vi "LTE Configure Common.vi"(0 "RFmx Handle In":refnum<k21>, 1 "Selector String":string, 5 "Common Configuration":T1={"Center Frequency (Hz)"=1000000000.0, "Reference Level (dBm)"=0.0, "External Attenuation (dB)"=0.0, "Trigger Enabled"=TRUE, "Digital Trigger Source"="PXI_Trig0", "Trigger Delay (s)"=0.0, "Selected Ports"=""} {"Trigger Delay (s)" format="%.2p"; "External Attenuation (dB)" format="%.2f"; "Reference Level (dBm)" format="%.2f"; "Center Frequency (Hz)" format="%.6p"}, 11 "error in (no error)":errorcluster) -> (4 "RFmx Handle Out":refnum<k21>, 15 "error out":errorcluster)   [LabVIEW 2016, in "RFmxLTE.lvlib"]
uses:
  RFmxLTE.lvlib
  Common/SA Common Configuration.ctl
  <vilib>/RFmx/LTE/mx/RFmxLTE.llb/RFmxLTE Configure Digital Edge Trigger.vi
  <resource>/objmgr/RFmxLTE.rc
  Common/Common.lvlib
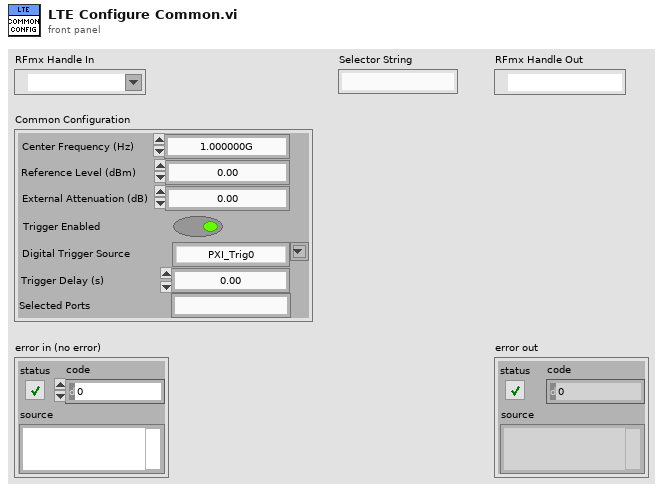
[diagram p1: front panel]
types:
  T1 = typedef "Common.lvlib/SA Common Configuration.ctl" = cluster{"Center Frequency (Hz)":dbl, "Reference Level (dBm)":dbl, "External Attenuation (dB)":dbl, "Trigger Enabled":bool, "Digital Trigger Source":string, "Trigger Delay (s)":dbl, "Selected Ports":string}
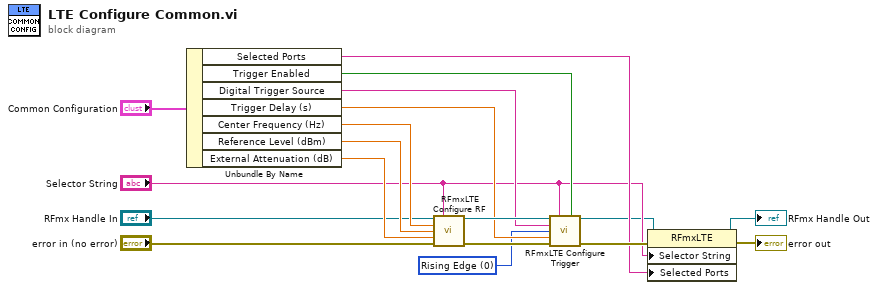
[diagram p0: block diagram]
diagram:
  w5 = 0 items=["Rising Edge", "Falling Edge"] ("Digital Edge")
  n1 = Unbundle By Name("Common Configuration") -> ("Selected Ports"=w3:string, "Trigger Enabled"=w9:bool, "Digital Trigger Source"=w11:string, "Trigger Delay (s)"=w10:dbl, "Center Frequency (Hz)"=w14:dbl, "Reference Level (dBm)"=w15:dbl, "External Attenuation (dB)"=w16:dbl)
  n2 = call <vilib>:"RFmxLTE Configure RF.vi"("Instrument Handle In"="RFmx Handle In", "Selector String"="Selector String", "Center Frequency (Hz)"=w14, "Reference Level"=w15, "External Attenuation (dB)"=w16, "error in (no error)"="error in (no error)") -> ("Instrument Handle Out"=w13:refnum<k21>, "error out"=w12:errorcluster)  [unwired: 8 in]
  n3 = call-poly <vilib>:"RFmxLTE Configure Trigger.vi"("Instrument Handle In"=w13, "Selector String"="Selector String", "Enable Trigger?"=w9, "Digital Edge Source"=w11, "Digital Edge"=w5, "Trigger Delay (s)"=w10, "error in (no error)"=w12) -> ("Instrument Handle Out"=w1:refnum<k21>, "error out"=w7:errorcluster)  [unwired: 7 in]
  n4 = property class="RFmxLTE"(reference=w1, error in=w7, "Selector String"="Selector String", "Selected Ports"=w3) -> (reference out=→"RFmx Handle Out":refnum<k21>, error out=→"error out":errorcluster)
